vi "400MHz Open Session.vi"(8 "error in (no error)":errorcluster, 10 "Input":T1={"MICS_ID"=0, "Use Local"=FALSE, "MICS Channel"=2} {"MICS_ID" step=1 format="%06x"}, 11 "MICS Dongle Address":refnum<visa-resource-name>="COM5") -> (0 "error out":errorcluster, 2 "Response":string)   [LabVIEW 2010]
uses:
  MICS_ID Global.vi
  MICS_Channel Global.vi
  <vilib>/Instr/_visa.llb/VISA Configure Serial Port (Instr).vi
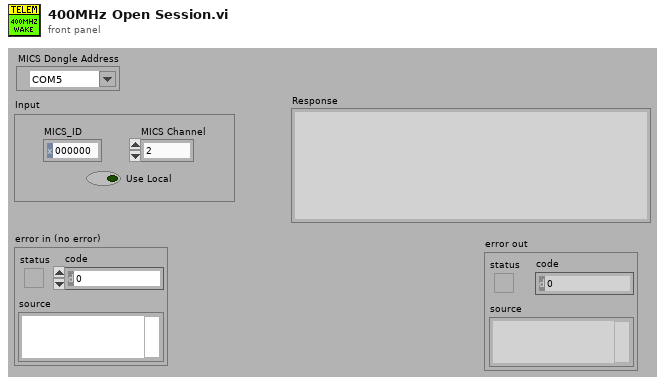
[diagram p1: front panel]
types:
  T1 = cluster{"MICS_ID":u32, "Use Local":bool, "MICS Channel":u16}
  T2 = cluster{"ConfigFlags":u8, "ImplantID":u32, "CompanyID":u8, "Normal_Comm":cluster{"RF_Channel":u8, "UserData":u8, "TX_Mod":u8, "RX_Mod":u8, "RX_BlockSize":u8, "BlockPerPack":u8, "TX_BlockSize":u8}, "Emerg_Comm":cluster{"RF_Channel":u8, "UserData":u8, "TX_Mod":u8, "RX_Mod":u8, "TX_BlockSize":u8, "BlockPerPack":u8, "RX_BlockSize":u8}, "ImplantRev":u8, "245TX_PowerCal":i8, "245TX_Power":i8, "CCA_RSSI_Thresholds":cluster{"ch0":u16, "ch1":u16, "ch2":u16, "ch3":u16, "ch4":u16, "ch5":u16, "ch6":u16, "ch7":u16, "ch8":u16, "ch9":u16}}
  T3 = cluster{"ERROR_OCCURRED":bool, "LINK_STAT_CHANGED":bool, "LINK_QUAL_CHANGED":bool, "400MHZ_TX_ACTIVE":bool, "400MHZ_RX_ACTIVE":bool, "245GHZ_TX_ACTIVE":bool, "DATA_STAT_CHANGED":bool, "SLEEPING":bool, "IDLE":bool, "SEARCHING_FOR_IMPLANT":bool, "STARTING_SESSION":bool, "LISTENING_FOR_EMERG":bool, "IN_SESSION":bool}
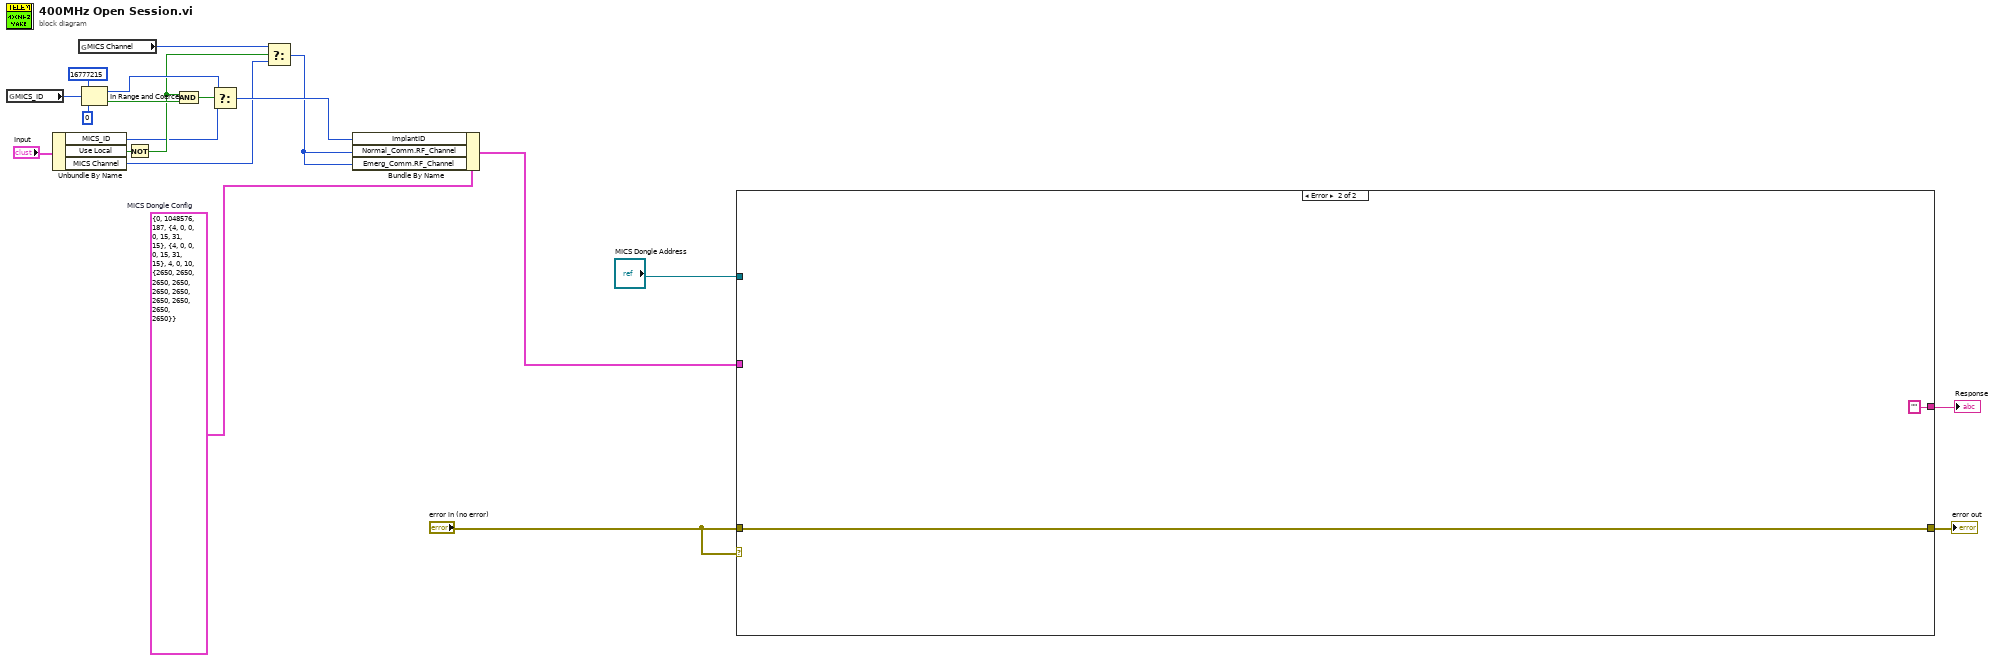
[diagram p0: block diagram]
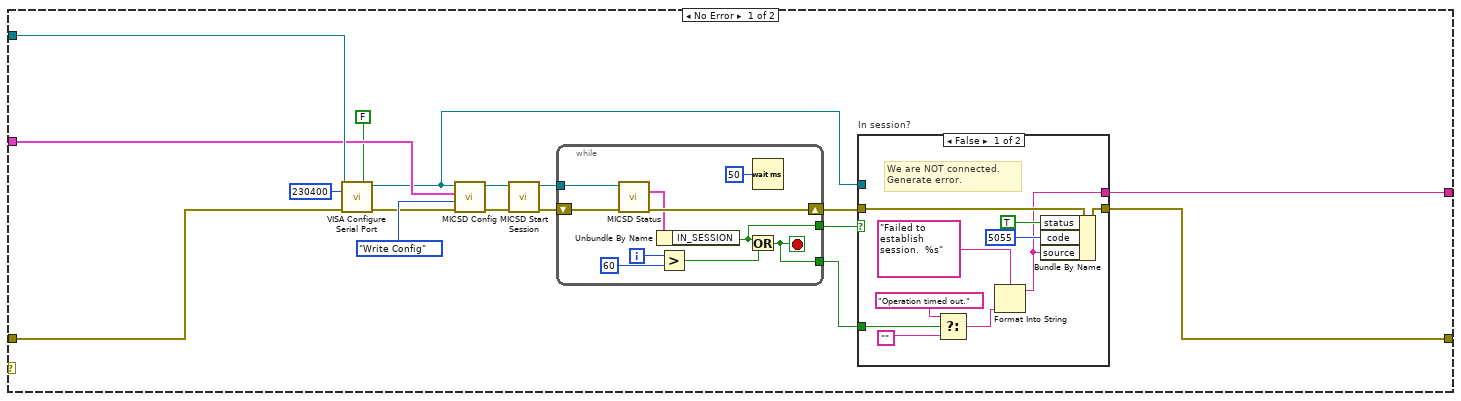
[diagram p2: hidden frame]
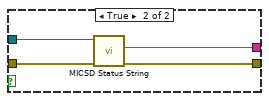
[diagram p3: hidden frame]
diagram:
  w12 = T2 {"ConfigFlags"=0, "ImplantID"=1048576, "CompanyID"=187, "Normal_Comm"={"RF_Channel"=4, "UserData"=0, "TX_Mod"=0, "RX_Mod"=0, "RX_BlockSize"=15, "BlockPerPack"=31, "TX_BlockSize"=15}, "Emerg_Comm"={"RF_Channel"=4, "UserData"=0, "TX_Mod"=0, "RX_Mod"=0, "TX_BlockSize"=15, "BlockPerPack"=31, "RX_BlockSize"=15}, "ImplantRev"=4, "245TX_PowerCal"=0, "245TX_Power"=10, "CCA_RSSI_Thresholds"={"ch0"=2650, "ch1"=2650, "ch2"=2650, "ch3"=2650, "ch4"=2650, "ch5"=2650, "ch6"=2650, "ch7"=2650, "ch8"=2650, "ch9"=2650}}  # MICS Dongle Config
  n1 = global read "MICS_ID Global.vi" "MICS_ID"() -> (w20:u32)
  n2 = Unbundle By Name("Input") -> ("MICS_ID"=w7:u32, "Use Local"=w8:bool, "MICS Channel"=w1:u16)
  n3 = global read "MICS_Channel Global.vi" "MICS Channel"() -> (w14:u16)
  n4 = In Range and Coerce(upper limit=u32 16777215, x=w20, lower limit=u32 0) -> (coerced(x)=w15:u32, In Range?=w17:bool)
  n5 = Not(x=w8) -> (.not. x?=w13:bool)
  n6 = And(x=w13, y=w17) -> (x .and. y?=w16:bool)
  n7 = Select(t=w15, s=w16, f=w7) -> (s? t:f=w10:u32)
  n8 = Select(t=w14, s=w13, f=w1) -> (s? t:f=w9:u16)
  n9 = Bundle By Name(cluster=w12, "ImplantID"=w10, "Normal_Comm.RF_Channel"=w9, "Emerg_Comm.RF_Channel"=w9) -> (w11:T2)
  n10 = case shown="Error" "error in (no error)" {
    tunnel: "error in (no error)" -> [w37 w63]
    tunnel: [w36 w63] -> w5
    tunnel: "MICS Dongle Address" -> [w35 _]
    tunnel: w11 -> [w34 _]
    tunnel: [w21 "" ("Response")] -> w3
    frame No Error {
      n11 = call-poly "VISA Configure Serial Port"("VISA resource name"=w35, "Enable Termination\nChar (T)"=FALSE ("Enable Termination\nChar (T)"), "baud rate (9600)"=u32 230400, "error in (no error)"=w37) -> ("VISA resource name out"=w22:refnum<visa-resource-name>, "error out"=w23:errorcluster)  [unwired: 10 in]
      n12 = call "MICSD Config.vi"("error in (no error)"=w23, "Function"=enum16{"Write Config", "Read Config"}."Write Config", "MICS_Config_In"=w34, "VISA Resource Name"=w22) -> ("error out"=w32:errorcluster, "dup VISA Resource Name"=w31:refnum<visa-resource-name>)  [unwired: 5 in, 1 out]
      n13 = call "MICSD Start Session.vi"("error in (no error)"=w32, "VISA Resource Name"=w31) -> ("error out"=w30:errorcluster, "dup VISA Resource Name"=w29:refnum<visa-resource-name>)  [unwired: 8 in]
      n14 = while {
        tunnel: w29 -> [w60]
        shift-right: [w59] -> w27
        shift-left: w30 -> [w61]
        tunnel: [w53] -> w28
        tunnel: [w52] -> w26
        i -> [w55]
        stop <- w52 stop-if-true
        n15 = call "MICSD Status.vi"("VISA Resource Name"=w60, "error in (no error)"=w61) -> ("Status Flags"=w58:T3, "error out"=w59:errorcluster)  [unwired: 7 in, 5 out]
        n16 = Unbundle By Name(w58) -> ("IN_SESSION"=w53:bool)
        n17 = Greater?(x=w55, y=60) -> (0:w56:bool)
        n18 = Or(x=w53, y=w56) -> (x .or. y?=w52:bool)
        n19 = Wait (ms)(milliseconds to wait=u32 50) -> ()  [unwired: 1 out]
      }
      n20 = case "In session?" shown="False" w28 {
        tunnel: w27 -> [w47 w51]
        tunnel: [w41 w50] -> w36
        tunnel: w26 -> [w45 _]
        tunnel: w22 -> [_ w49]
        tunnel: [w38 w48] -> w21
        frame False {
          # "We are NOT connected. Generate error."
          n21 = Select(t="Operation timed out." ("format string"), s=w45, f="") -> (s? t:f=w40:string)
          n22 = Format Into String(format string="Failed to establish session.  %s", w40) -> (resulting string=w38:string)  [unwired: 2 in, 1 out]
          n23 = Bundle By Name(cluster=w47, "status"=TRUE, "code"=5055, "source"=w38) -> (w41:errorcluster)
        }
        frame True {
          n24 = call "MICSD Status String.vi"("error in (no error)"=w51, "VISA Resource Name"=w49) -> ("error out"=w50:errorcluster, "Response"=w48:string)  [unwired: 7 in, 1 out]
        }
      }
    }
    frame Error {
      (unwired) ""
    }
  }
  "error out" <- w5
  "Response" <- w3
